vi "220613 VNA DATA TO AVG.vi"(3 "Array of SD to average":T2(array[cluster])) -> (1 "AVERAGED SD":T1)   [LabVIEW 2021]
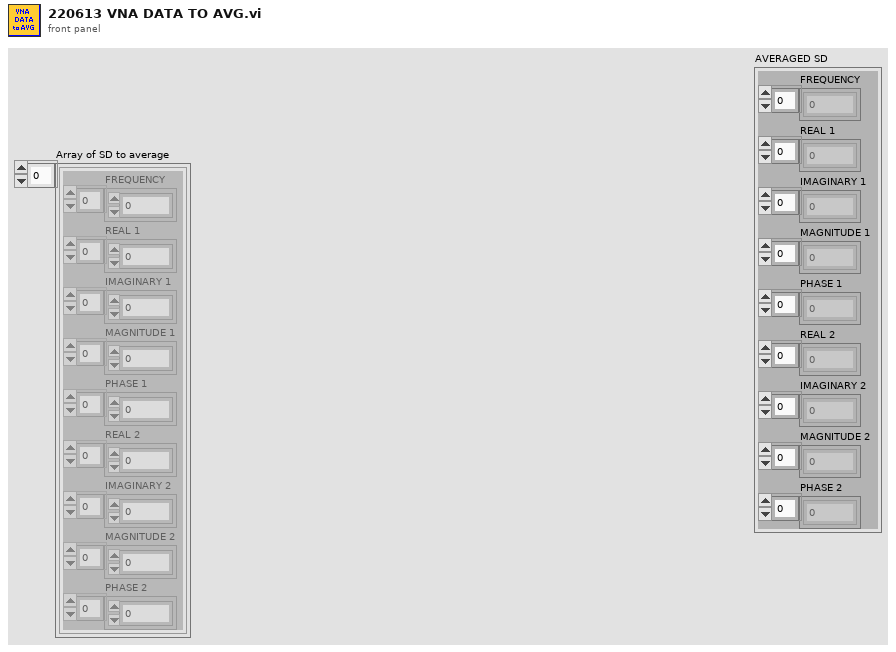
[diagram p1: front panel]
types:
  T1 = cluster{"FREQUENCY":sgl[], "REAL 1":dbl[], "IMAGINARY 1":sgl[], "MAGNITUDE 1":dbl[], "PHASE 1":dbl[], "REAL 2":dbl[], "IMAGINARY 2":sgl[], "MAGNITUDE 2":dbl[], "PHASE 2":dbl[]}
  T2 = cluster{"FREQUENCY":sgl[], "REAL 1":dbl[], "IMAGINARY 1":sgl[], "MAGNITUDE 1":dbl[], "PHASE 1":dbl[], "REAL 2":dbl[], "IMAGINARY 2":sgl[], "MAGNITUDE 2":dbl[], "PHASE 2":dbl[]}[]
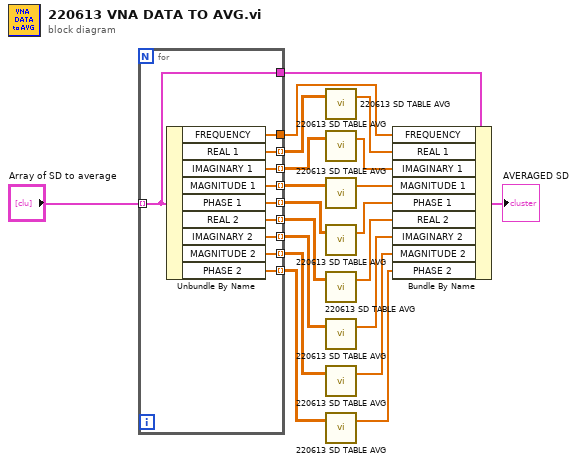
[diagram p0: block diagram]
diagram:
  n1 = for {
    tunnel: "Array of SD to average" -> [w21] mode=indexing
    tunnel: [w30] -> w19 mode=indexing
    tunnel: [w29] -> w18 mode=indexing
    tunnel: [w28] -> w10
    tunnel: [w27] -> w17 mode=indexing
    tunnel: [w26] -> w16 mode=indexing
    tunnel: [w25] -> w15 mode=indexing
    tunnel: [w24] -> w14 mode=indexing
    tunnel: [w23] -> w13 mode=indexing
    tunnel: [w22] -> w12 mode=indexing
    tunnel: [w21] -> w11
    n2 = Unbundle By Name(w21) -> ("FREQUENCY"=w28:sgl[], "REAL 1"=w30:dbl[], "IMAGINARY 1"=w29:sgl[], "MAGNITUDE 1"=w27:dbl[], "PHASE 1"=w26:dbl[], "REAL 2"=w25:dbl[], "IMAGINARY 2"=w24:sgl[], "MAGNITUDE 2"=w23:dbl[], "PHASE 2"=w22:dbl[])
  }
  n3 = call "220613 SD TABLE AVG.vi"("Table of SD to average"=w19) -> ("Average SD"=w9:dbl[])  [unwired: 2 in]
  n4 = call "220613 SD TABLE AVG.vi"("Table of SD to average"=w18) -> ("Average SD"=w8:dbl[])  [unwired: 2 in]
  n5 = call "220613 SD TABLE AVG.vi"("Table of SD to average"=w17) -> ("Average SD"=w7:dbl[])  [unwired: 2 in]
  n6 = call "220613 SD TABLE AVG.vi"("Table of SD to average"=w16) -> ("Average SD"=w6:dbl[])  [unwired: 2 in]
  n7 = call "220613 SD TABLE AVG.vi"("Table of SD to average"=w15) -> ("Average SD"=w5:dbl[])  [unwired: 2 in]
  n8 = call "220613 SD TABLE AVG.vi"("Table of SD to average"=w14) -> ("Average SD"=w4:dbl[])  [unwired: 2 in]
  n9 = call "220613 SD TABLE AVG.vi"("Table of SD to average"=w13) -> ("Average SD"=w3:dbl[])  [unwired: 2 in]
  n10 = call "220613 SD TABLE AVG.vi"("Table of SD to average"=w12) -> ("Average SD"=w2:dbl[])  [unwired: 2 in]
  n11 = Bundle By Name(cluster=w11, "FREQUENCY"=w10, "REAL 1"=w9, "IMAGINARY 1"=w8, "MAGNITUDE 1"=w7, "PHASE 1"=w6, "REAL 2"=w5, "IMAGINARY 2"=w4, "MAGNITUDE 2"=w3, "PHASE 2"=w2) -> (→"AVERAGED SD":T1)
